vi "SavedSettingsSplitDescription.vi"(11 "Description in":string) -> (2 "Options":T1, 3 "Description out":string)   [LabVIEW 2021]
uses:
  SavedSettingsOptions.ctl
  <vilib>/regexp/Match Regular Expression.xnode
panel:
  in  "Options dummy":T1
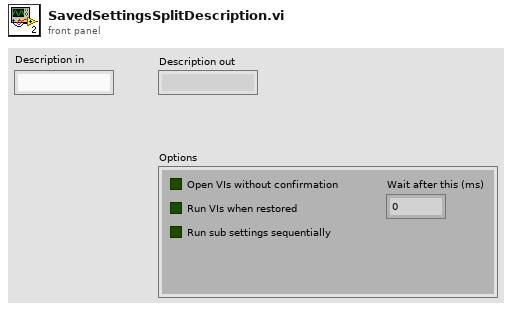
[diagram p1: front panel]
types:
  T1 = typedef "SavedSettingsOptions.ctl" = cluster{"OpenVIs":bool, "RunVIs":bool, "RestoreSubItems":bool, "WaitAfter":u32}
  T2 = cluster{"Type":enum16{"null", "number", "boolean", "string", "array", "object", ""}, "Value":variant}
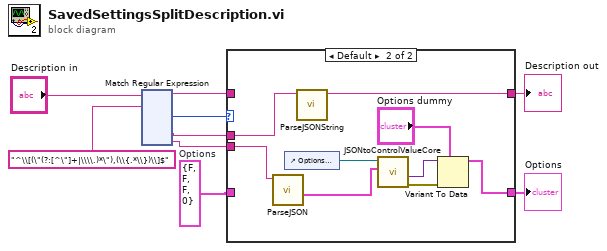
[diagram p0: block diagram]
diagram:
  w2 = T1 {"OpenVIs"=FALSE, "RunVIs"=FALSE, "RestoreSubItems"=FALSE, "WaitAfter"=0}  # Options
  n1 = xnode "Match Regular Expression"("input string"="Description in", "regular expression"="^\\[(\"(?:[^\"]+|\\\\.)*\"),(\\{.*\\})\\]$") -> ("before match"=w6:string, "offset past match"=w7:i32, "submatch 1"=w5:string, "submatch 2"=w4:string)  [unwired: 4 in, 3 out]
  n2 = case shown="Default" w7 {
    tunnel: w6 -> [w11 _]
    tunnel: [w11 w19] -> w3
    tunnel: w2 -> [w10 _]
    tunnel: [w10 w14] -> w1
    tunnel: w5 -> [_ w20]
    tunnel: w4 -> [_ w18]
    frame -1 {
    }
    frame Default {
      n3 = call "ParseJSON.vi"("JSON string"=w18) -> ("Value"=w17:T2)  [unwired: 6 in, 4 out]
      n4 = control-ref of="Options dummy"() -> (w12:refnum<vi>)
      n5 = call "ParseJSONString.vi"("JSON string"=w20) -> ("string"=w19:string)  [unwired: 9 in, 1 out]
      n6 = call "JSONtoControlValueCore.vi"("Value"=w17, "Control in"=w12) -> ("error out"=w16:errorcluster, "Variant"=w15:variant)  [unwired: 8 in]
      n7 = Variant To Data(error in=w16, type="Options dummy", Variant=w15) -> (data=w14:T1)  [unwired: 1 out]
    }
  }
  "Description out" <- w3
  "Options" <- w1
